vi "OP5_PRESSURIZZAZIONE.vi"(0 "Esito 2 in":cluster{"Si":bool, "No":bool}, 1 "Esito 3 in":cluster{"Si":bool, "No":bool}, 2 "Esito 4 in":cluster{"Si":bool, "No":bool}, 3 "Esito 5 in":cluster{"Si":bool, "No":bool}, 4 "Esito 6 in":cluster{"Si":bool, "No":bool}, 5 "Esito 7 in":cluster{"Si":bool, "No":bool}, 6 "Esito 8 in":cluster{"Si":bool, "No":bool}, 7 "Esito 9 in":cluster{"Si":bool, "No":bool}, 8 "Esito 1 in":cluster{"Si":bool, "No":bool}, 9 "Tasto premuto":T1(array[ring]), 10 "Tipo specifica":string, 12 "Stato in":u16, 14 "Stato out":u16) -> (16 "Dato":string[](array[string]), 17 "ANNULLA PROVA":bool, 18 "Esito 1 out":T2, 19 "i out":i32=1, 20 "Esito 2 out":T2, 21 "Esito 3 out":T2, 22 "Esito 4 out":T2, 23 "Esito 5 out":T2, 24 "Esito 6 out":T2, 25 "Esito 7 out":T2, 26 "Esito 8 out":T2, 27 "Esito 9 out":T2)   [LabVIEW 2022 SP3]
uses:
  Labview/Globali.vi
panel:
  in  "i max":i32
  in  "i":i32=1
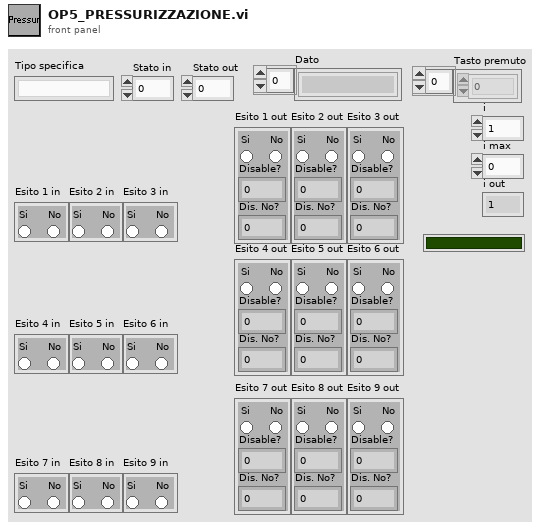
[diagram p1: front panel]
types:
  T1 = enum16{"0", "1", "2", "3", "4", "5", "6", "7", "8", "9", "A", "B", "C", "D", "E", "F", "G", "H", "I", "J", "K", "L", "M", "N", "O", "P", "Q", "R", "S", "T", "U", "V", "W", "X", "Y", "Z", "F1", "F2", "F3", "F4", "F5", "F6", "F7", "F8", "F9", "F10", "F11", "F12", "F13", "F14", "F15", "ADD", "BACK", "BACKSLASH", "CAPITAL", "COMMA", "DECIMAL", "DELETE", "DIVIDE", "DOWN", "END", "EQUALS", "ESCAPE", "GRAVE (`)", "HOME", "INSERT", "LBRACKET", "LCONTROL", "LEFT", "L ALT", "LSHIFT", "LWIN", "MINUS", "MULTIPLY", "NEXT", "NUMLOCK", "NUMPAD_0", "NUMPAD_1", "NUMPAD_2", "NUMPAD_3", "NUMPAD_4", "NUMPAD_5", "NUMPAD_6", "NUMPAD_7", "NUMPAD_8", "NUMPAD_9", "PAUSE", "PERIOD", "PRIOR (PG UP)", "RBRACKET", "RCONTROL", "RETURN", "RIGHT", "R ALT", "RSHIFT", "RWIN", "SCROLL", "SEMICOLON", "SLASH", "SPACE", "SUBTRACT", "TAB", "UP", "ENTER (num pad)", "' (quote)"}[]
  T2 = cluster{"Disable?":i16, "Si":bool, "No":bool, "Dis. No?":i16}
  T3 = cluster{"Esito 1 out":cluster{"Disable?":i16, "Si":bool, "No":bool, "Dis. No?":i16}, "Esito 2 out":cluster{"Disable?":i16, "Si":bool, "No":bool, "Dis. No?":i16}, "Esito 3 out":cluster{"Disable?":i16, "Si":bool, "No":bool, "Dis. No?":i16}, "Esito 4 out":cluster{"Disable?":i16, "Si":bool, "No":bool, "Dis. No?":i16}, "Esito 5 out":cluster{"Disable?":i16, "Si":bool, "No":bool, "Dis. No?":i16}, "Esito 6 out":cluster{"Disable?":i16, "Si":bool, "No":bool, "Dis. No?":i16}, "Esito 7 out":cluster{"Disable?":i16, "Si":bool, "No":bool, "Dis. No?":i16}, "Esito 8 out":cluster{"Disable?":i16, "Si":bool, "No":bool, "Dis. No?":i16}, "Esito 9 out":cluster{"Disable?":i16, "Si":bool, "No":bool, "Dis. No?":i16}}
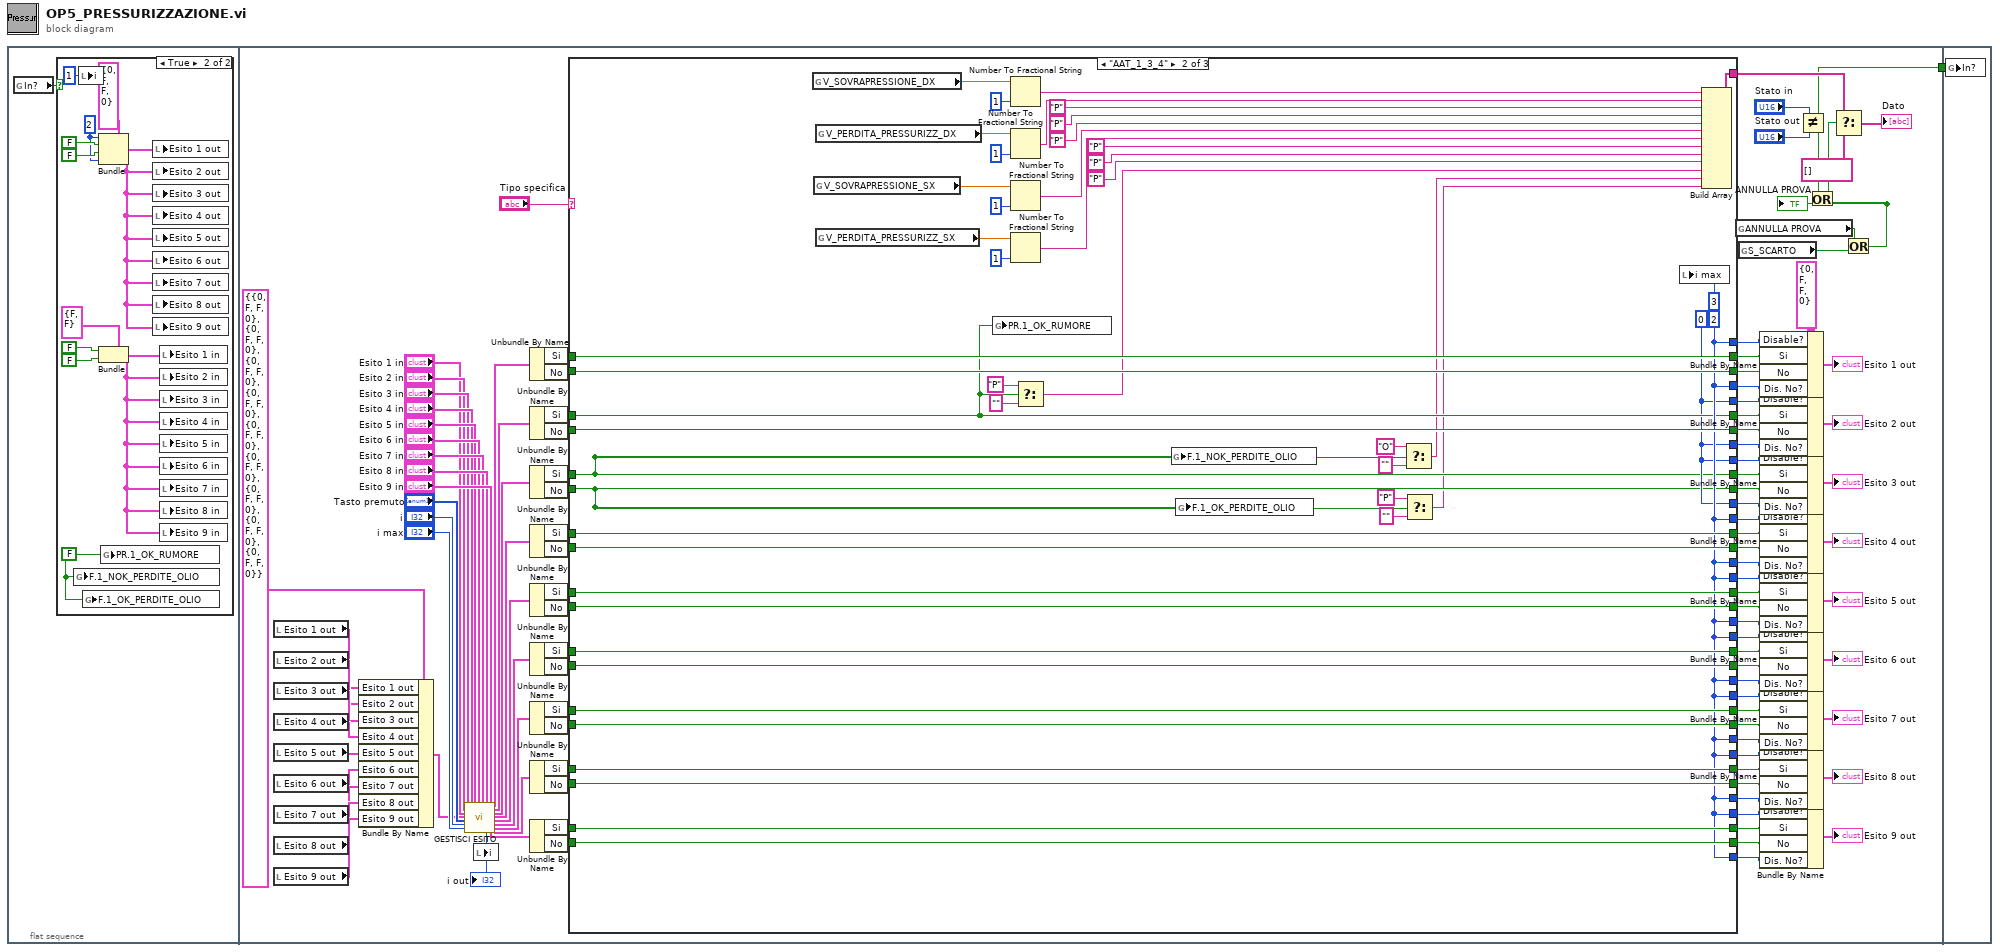
[diagram p0: block diagram]
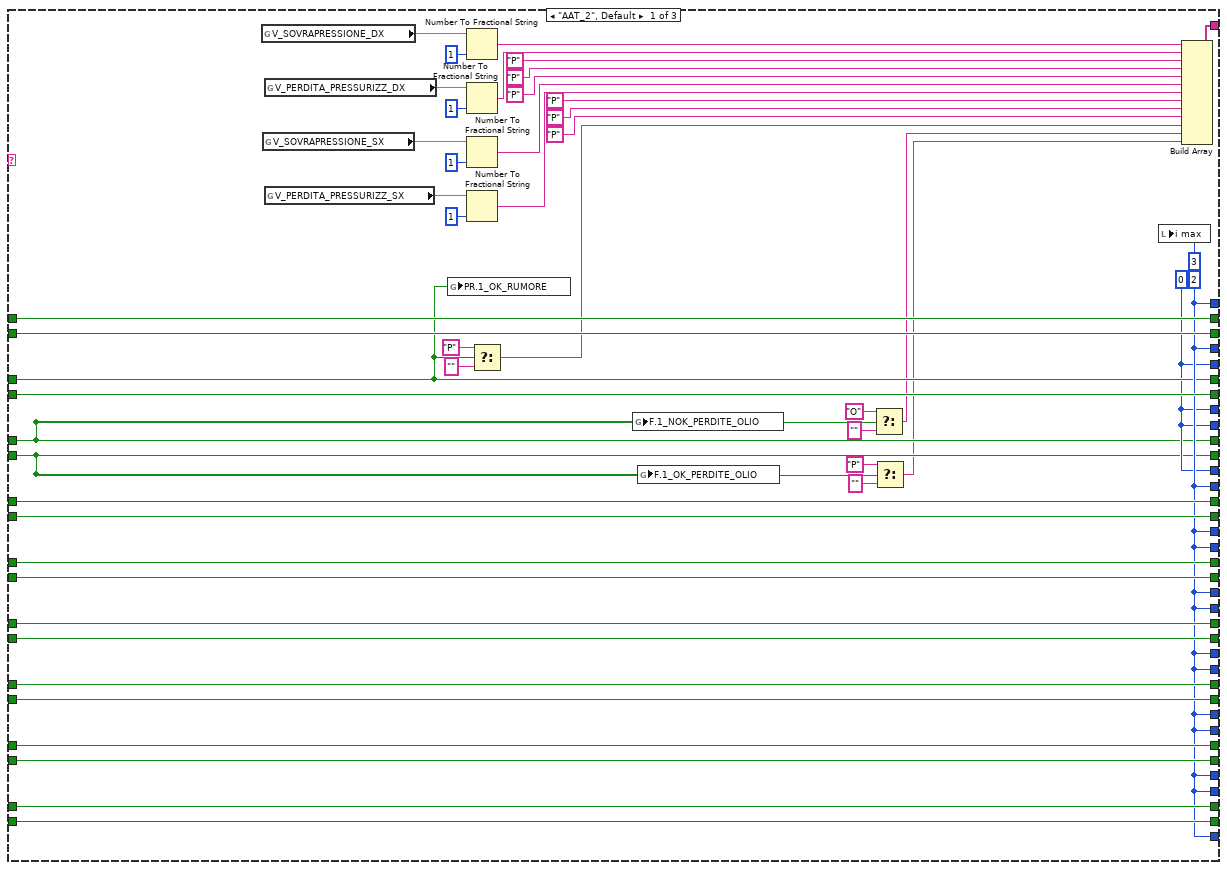
[diagram p3: hidden frame]
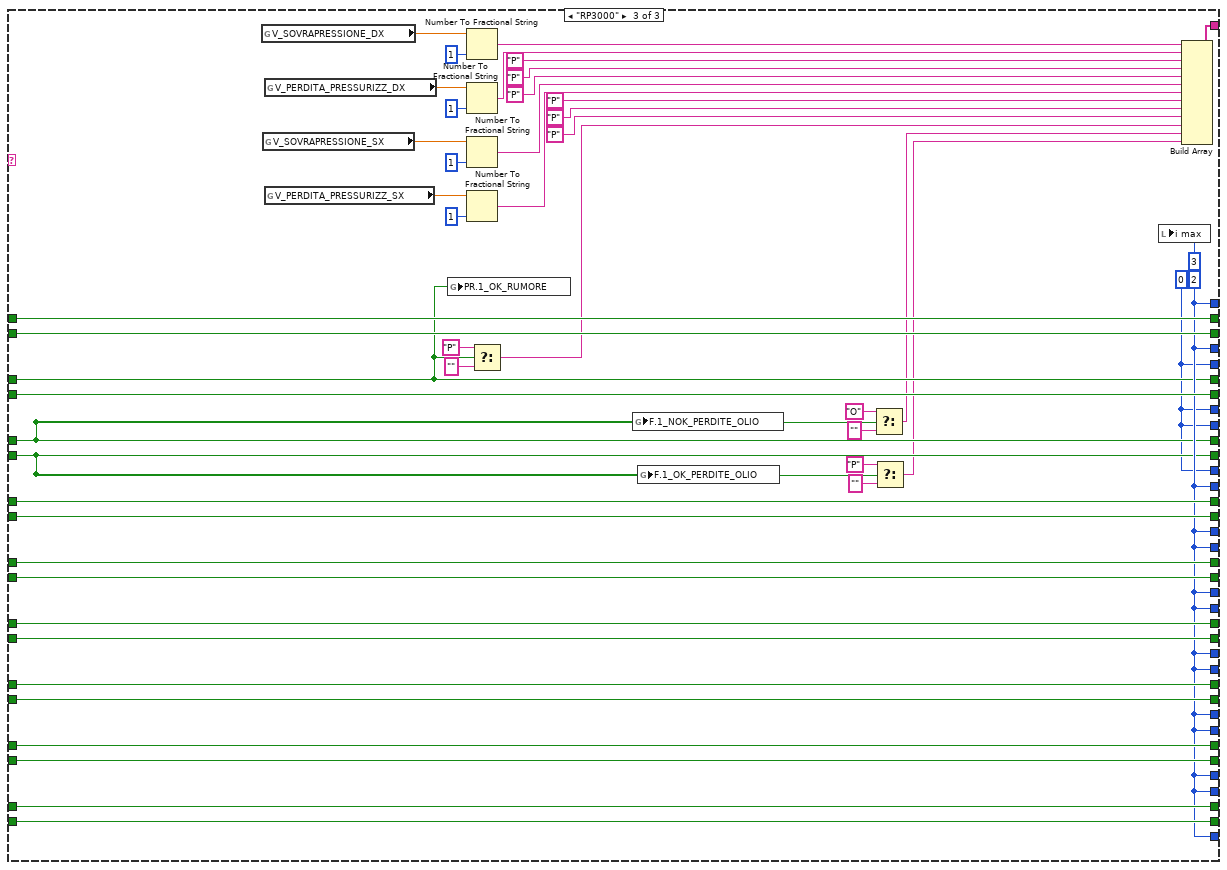
[diagram p4: hidden frame]
diagram:
  n1 = flat-sequence {
    tunnel: [w18] -> w1
    tunnel: w1 -> [w269]
    frame #0 {
      n2 = global read "Globali.vi" "In?"() -> (w2:bool)
      n3 = case shown="True" w2 {
        frame False {
        }
        frame True {
          w3 = FALSE ("No")
          w10 = i16 2 ("Disable?")
          n4 = global write "Globali.vi" "F.1_NOK_PERDITE_OLIO"(w3) -> ()
          n5 = local write "i"(1 ("i")) -> ()
          n6 = global write "Globali.vi" "F.1_OK_PERDITE_OLIO"(w3) -> ()
          n7 = Bundle(cluster=T2 {"Disable?"=0, "Si"=FALSE, "No"=FALSE, "Dis. No?"=0} ("Esito 1 out"), "Disable?"=w10, "Si"=FALSE, "No"=FALSE, "Dis. No?"=w10) -> (w9:T2)
          n8 = Bundle(cluster=cluster{"Si":bool, "No":bool} {"Si"=FALSE, "No"=FALSE} ("Esito 1 in"), "Si"=FALSE, "No"=FALSE) -> (w7:cluster{"Si":bool, "No":bool})
          n9 = global write "Globali.vi" "PR.1_OK_RUMORE"(w3) -> ()
          n10 = local write "Esito 1 out"(w9) -> ()
          n11 = local write "Esito 2 out"(w9) -> ()
          n12 = local write "Esito 3 out"(w9) -> ()
          n13 = local write "Esito 4 out"(w9) -> ()
          n14 = local write "Esito 5 out"(w9) -> ()
          n15 = local write "Esito 6 out"(w9) -> ()
          n16 = local write "Esito 7 out"(w9) -> ()
          n17 = local write "Esito 8 out"(w9) -> ()
          n18 = local write "Esito 9 out"(w9) -> ()
          n19 = local write "Esito 1 in"(w7) -> ()
          n20 = local write "Esito 2 in"(w7) -> ()
          n21 = local write "Esito 3 in"(w7) -> ()
          n22 = local write "Esito 4 in"(w7) -> ()
          n23 = local write "Esito 5 in"(w7) -> ()
          n24 = local write "Esito 6 in"(w7) -> ()
          n25 = local write "Esito 7 in"(w7) -> ()
          n26 = local write "Esito 8 in"(w7) -> ()
          n27 = local write "Esito 9 in"(w7) -> ()
        }
      }
    }
    frame #1 {
      w61 = T2 {"Disable?"=0, "Si"=FALSE, "No"=FALSE, "Dis. No?"=0} ("Esito 1 out")
      n28 = local read "Esito 1 out"() -> (w39:T2)
      n29 = local read "Esito 2 out"() -> (w40:T2)
      n30 = local read "Esito 3 out"() -> (w41:T2)
      n31 = local read "Esito 4 out"() -> (w42:T2)
      n32 = local read "Esito 5 out"() -> (w43:T2)
      n33 = local read "Esito 6 out"() -> (w44:T2)
      n34 = local read "Esito 7 out"() -> (w45:T2)
      n35 = local read "Esito 8 out"() -> (w46:T2)
      n36 = local read "Esito 9 out"() -> (w47:T2)
      n37 = Bundle By Name(cluster=T3 {"Esito 1 out"={"Disable?"=0, "Si"=FALSE, "No"=FALSE, "Dis. No?"=0}, "Esito 2 out"={"Disable?"=0, "Si"=FALSE, "No"=FALSE, "Dis. No?"=0}, "Esito 3 out"={"Disable?"=0, "Si"=FALSE, "No"=FALSE, "Dis. No?"=0}, "Esito 4 out"={"Disable?"=0, "Si"=FALSE, "No"=FALSE, "Dis. No?"=0}, "Esito 5 out"={"Disable?"=0, "Si"=FALSE, "No"=FALSE, "Dis. No?"=0}, "Esito 6 out"={"Disable?"=0, "Si"=FALSE, "No"=FALSE, "Dis. No?"=0}, "Esito 7 out"={"Disable?"=0, "Si"=FALSE, "No"=FALSE, "Dis. No?"=0}, "Esito 8 out"={"Disable?"=0, "Si"=FALSE, "No"=FALSE, "Dis. No?"=0}, "Esito 9 out"={"Disable?"=0, "Si"=FALSE, "No"=FALSE, "Dis. No?"=0}} ("Cluster"), "Esito 1 out"=w39, "Esito 2 out"=w40, "Esito 3 out"=w41, "Esito 4 out"=w42, "Esito 5 out"=w43, "Esito 6 out"=w44, "Esito 7 out"=w45, "Esito 8 out"=w46, "Esito 9 out"=w47) -> (w48:T3)
      n38 = call "GESTISCI ESITO.vi"("Esito 3 in"="Esito 3 in", "Esito 2 in"="Esito 2 in", "Esito 1 in"="Esito 1 in", "Cluster"=w48, "Tasto premuto"="Tasto premuto", "i in"="i", "i max"="i max", "Esito 4 in"="Esito 4 in", "Esito 5 in"="Esito 5 in", "Esito 6 in"="Esito 6 in", "Esito 7 in"="Esito 7 in", "Esito 8 in"="Esito 8 in", "Esito 9 in"="Esito 9 in") -> ("i out"=w19:i32, "Esito 9 in 2"=w37:cluster{"Si":bool, "No":bool}, "Esito 1 in 2"=w29:cluster{"Si":bool, "No":bool}, "Esito 2 in 2"=w30:cluster{"Si":bool, "No":bool}, "Esito 3 in 2"=w31:cluster{"Si":bool, "No":bool}, "Esito 4 in 2"=w32:cluster{"Si":bool, "No":bool}, "Esito 5 in 2"=w33:cluster{"Si":bool, "No":bool}, "Esito 6 in 2"=w34:cluster{"Si":bool, "No":bool}, "Esito 7 in 2"=w36:cluster{"Si":bool, "No":bool}, "Esito 8 in 2"=w35:cluster{"Si":bool, "No":bool})  [unwired: 5 in]
      "i out" <- w19
      n39 = local write "i"(w19) -> ()
      n40 = Unbundle By Name(w29) -> ("Si"=w85:bool, "No"=w84:bool)
      n41 = Unbundle By Name(w30) -> ("Si"=w68:bool, "No"=w69:bool)
      n42 = Unbundle By Name(w31) -> ("Si"=w70:bool, "No"=w71:bool)
      n43 = Unbundle By Name(w32) -> ("Si"=w72:bool, "No"=w73:bool)
      n44 = Unbundle By Name(w33) -> ("Si"=w74:bool, "No"=w75:bool)
      n45 = Unbundle By Name(w34) -> ("Si"=w76:bool, "No"=w77:bool)
      n46 = Unbundle By Name(w36) -> ("Si"=w78:bool, "No"=w79:bool)
      n47 = Unbundle By Name(w35) -> ("Si"=w80:bool, "No"=w81:bool)
      n48 = Unbundle By Name(w37) -> ("Si"=w82:bool, "No"=w83:bool)
      n49 = case shown="\"AAT_1_3_4\"" "Tipo specifica" {
        tunnel: [w148 w193 w246] -> w65
        tunnel: [w155 w204 w253] -> w112
        tunnel: [w130 w179 w224] -> w111
        tunnel: [w130 w179 w224] -> w110
        tunnel: [w155 w204 w253] -> w109
        tunnel: [w155 w204 w253] -> w108
        tunnel: [w155 w204 w253] -> w107
        tunnel: [w155 w204 w253] -> w106
        tunnel: [w155 w204 w253] -> w105
        tunnel: [w155 w204 w253] -> w104
        tunnel: [w156 w205 w254] -> w103
        tunnel: [w161 w210 w259] -> w102
        tunnel: [w131 w180 w233] -> w101
        tunnel: [w162 w211 w260] -> w100
        tunnel: [w125 w174 w228] -> w99
        tunnel: [w124 w173 w227] -> w98
        tunnel: [w157 w206 w255] -> w97
        tunnel: [w170 w219 w268] -> w96
        tunnel: [w160 w209 w258] -> w95
        tunnel: [w169 w218 w267] -> w94
        tunnel: [w159 w208 w257] -> w93
        tunnel: [w168 w217 w266] -> w92
        tunnel: [w158 w207 w256] -> w91
        tunnel: [w167 w216 w265] -> w90
        tunnel: [w166 w215 w264] -> w89
        tunnel: [w165 w214 w263] -> w88
        tunnel: [w164 w213 w262] -> w87
        tunnel: [w163 w212 w261] -> w86
        tunnel: w85 -> [w156 w205 w254]
        tunnel: w84 -> [w161 w210 w259]
        tunnel: w83 -> [w163 w212 w261]
        tunnel: w82 -> [w164 w213 w262]
        tunnel: w81 -> [w165 w214 w263]
        tunnel: w80 -> [w166 w215 w264]
        tunnel: w79 -> [w167 w216 w265]
        tunnel: w78 -> [w158 w207 w256]
        tunnel: w77 -> [w168 w217 w266]
        tunnel: w76 -> [w159 w208 w257]
        tunnel: w75 -> [w169 w218 w267]
        tunnel: w74 -> [w160 w209 w258]
        tunnel: w73 -> [w170 w219 w268]
        tunnel: w72 -> [w157 w206 w255]
        tunnel: w71 -> [w124 w173 w227]
        tunnel: w70 -> [w125 w174 w228]
        tunnel: w69 -> [w162 w211 w260]
        tunnel: w68 -> [w131 w180 w233]
        tunnel: [w155 w204 w253] -> w60
        tunnel: [w130 w179 w224] -> w59
        tunnel: [w130 w179 w224] -> w58
        tunnel: [w155 w204 w253] -> w57
        tunnel: [w155 w204 w253] -> w56
        tunnel: [w155 w204 w253] -> w55
        tunnel: [w155 w204 w253] -> w54
        tunnel: [w155 w204 w253] -> w53
        tunnel: [w155 w204 w253] -> w52
        frame "AAT_2", Default {
          w155 = 2
          w130 = 0
          n50 = global read "Globali.vi" "V_SOVRAPRESSIONE_DX"() -> (w135:sgl)
          n51 = global read "Globali.vi" "V_SOVRAPRESSIONE_SX"() -> (w133:sgl)
          n52 = global read "Globali.vi" "V_PERDITA_PRESSURIZZ_DX"() -> (w134:sgl)
          n53 = global read "Globali.vi" "V_PERDITA_PRESSURIZZ_SX"() -> (w132:sgl)
          n54 = global write "Globali.vi" "PR.1_OK_RUMORE"(w131) -> ()
          n55 = Number To Fractional String(number=w135, precision (6)=i16 1) -> (F-format string=w147:string)  [unwired: 2 in]
          n56 = Number To Fractional String(number=w134, precision (6)=i16 1) -> (F-format string=w146:string)  [unwired: 2 in]
          n57 = Number To Fractional String(number=w133, precision (6)=i16 1) -> (F-format string=w142:string)  [unwired: 2 in]
          n58 = Number To Fractional String(number=w132, precision (6)=i16 1) -> (F-format string=w141:string)  [unwired: 2 in]
          n59 = Select(t="P", s=w131, f="") -> (s? t:f=w137:string)
          n60 = global write "Globali.vi" "F.1_NOK_PERDITE_OLIO"(w125) -> ()
          n61 = global write "Globali.vi" "F.1_OK_PERDITE_OLIO"(w124) -> ()
          n62 = Select(t="O", s=w125, f="") -> (s? t:f=w123:string)
          n63 = Select(t="P", s=w124, f="") -> (s? t:f=w122:string)
          n64 = local write "i max"(3) -> ()
          n65 = Build Array(w147, w146, "P", "P", "P", w142, w141, "P", "P", "P", w137, w123, w122) -> (w148:string[])
        }
        frame "AAT_1_3_4" {
          w204 = 2
          w179 = 0
          n66 = global read "Globali.vi" "V_SOVRAPRESSIONE_DX"() -> (w199:sgl)
          n67 = global read "Globali.vi" "V_SOVRAPRESSIONE_SX"() -> (w196:sgl)
          n68 = global read "Globali.vi" "V_PERDITA_PRESSURIZZ_DX"() -> (w198:sgl)
          n69 = global read "Globali.vi" "V_PERDITA_PRESSURIZZ_SX"() -> (w197:sgl)
          n70 = global write "Globali.vi" "PR.1_OK_RUMORE"(w180) -> ()
          n71 = Number To Fractional String(number=w199, precision (6)=i16 1) -> (F-format string=w192:string)  [unwired: 2 in]
          n72 = Number To Fractional String(number=w198, precision (6)=i16 1) -> (F-format string=w191:string)  [unwired: 2 in]
          n73 = Number To Fractional String(number=w196, precision (6)=i16 1) -> (F-format string=w187:string)  [unwired: 2 in]
          n74 = Number To Fractional String(number=w197, precision (6)=i16 1) -> (F-format string=w186:string)  [unwired: 2 in]
          n75 = Select(t="P", s=w180, f="") -> (s? t:f=w182:string)
          n76 = global write "Globali.vi" "F.1_NOK_PERDITE_OLIO"(w174) -> ()
          n77 = global write "Globali.vi" "F.1_OK_PERDITE_OLIO"(w173) -> ()
          n78 = Select(t="O", s=w174, f="") -> (s? t:f=w172:string)
          n79 = Select(t="P", s=w173, f="") -> (s? t:f=w171:string)
          n80 = local write "i max"(3) -> ()
          n81 = Build Array(w192, w191, "P", "P", "P", w187, w186, "P", "P", "P", w182, w172, w171) -> (w193:string[])
        }
        frame "RP3000" {
          w253 = 2
          w224 = 0
          n82 = global read "Globali.vi" "V_SOVRAPRESSIONE_DX"() -> (w221:sgl)
          n83 = global read "Globali.vi" "V_SOVRAPRESSIONE_SX"() -> (w220:sgl)
          n84 = global read "Globali.vi" "V_PERDITA_PRESSURIZZ_DX"() -> (w222:sgl)
          n85 = global read "Globali.vi" "V_PERDITA_PRESSURIZZ_SX"() -> (w223:sgl)
          n86 = global write "Globali.vi" "PR.1_OK_RUMORE"(w233) -> ()
          n87 = Number To Fractional String(number=w221, precision (6)=i16 1) -> (F-format string=w245:string)  [unwired: 2 in]
          n88 = Number To Fractional String(number=w222, precision (6)=i16 1) -> (F-format string=w244:string)  [unwired: 2 in]
          n89 = Number To Fractional String(number=w220, precision (6)=i16 1) -> (F-format string=w240:string)  [unwired: 2 in]
          n90 = Number To Fractional String(number=w223, precision (6)=i16 1) -> (F-format string=w239:string)  [unwired: 2 in]
          n91 = Select(t="P", s=w233, f="") -> (s? t:f=w235:string)
          n92 = global write "Globali.vi" "F.1_NOK_PERDITE_OLIO"(w228) -> ()
          n93 = global write "Globali.vi" "F.1_OK_PERDITE_OLIO"(w227) -> ()
          n94 = Select(t="O", s=w228, f="") -> (s? t:f=w226:string)
          n95 = Select(t="P", s=w227, f="") -> (s? t:f=w225:string)
          n96 = local write "i max"(3) -> ()
          n97 = Build Array(w245, w244, "P", "P", "P", w240, w239, "P", "P", "P", w235, w226, w225) -> (w246:string[])
        }
      }
      n98 = global read "Globali.vi" "ANNULLA PROVA"() -> (w16:bool)
      n99 = global read "Globali.vi" "S_SCARTO"() -> (w15:bool)
      n100 = Bundle By Name(cluster=w61, "Disable?"=w112, "Si"=w103, "No"=w102, "Dis. No?"=w60) -> (→"Esito 1 out":T2)
      n101 = Bundle By Name(cluster=w61, "Disable?"=w111, "Si"=w101, "No"=w100, "Dis. No?"=w59) -> (→"Esito 2 out":T2)
      n102 = Bundle By Name(cluster=w61, "Disable?"=w110, "Si"=w99, "No"=w98, "Dis. No?"=w58) -> (→"Esito 3 out":T2)
      n103 = Bundle By Name(cluster=w61, "Disable?"=w109, "Si"=w97, "No"=w96, "Dis. No?"=w57) -> (→"Esito 4 out":T2)
      n104 = Bundle By Name(cluster=w61, "Disable?"=w108, "Si"=w95, "No"=w94, "Dis. No?"=w56) -> (→"Esito 5 out":T2)
      n105 = Bundle By Name(cluster=w61, "Disable?"=w107, "Si"=w93, "No"=w92, "Dis. No?"=w55) -> (→"Esito 6 out":T2)
      n106 = Bundle By Name(cluster=w61, "Disable?"=w106, "Si"=w91, "No"=w90, "Dis. No?"=w54) -> (→"Esito 7 out":T2)
      n107 = Bundle By Name(cluster=w61, "Disable?"=w105, "Si"=w89, "No"=w88, "Dis. No?"=w53) -> (→"Esito 8 out":T2)
      n108 = Bundle By Name(cluster=w61, "Disable?"=w104, "Si"=w87, "No"=w86, "Dis. No?"=w52) -> (→"Esito 9 out":T2)
      n109 = Not Equal?(x="Stato in", y="Stato out") -> (x != y?=w18:bool)
      n110 = Or(x=w16, y=w15) -> (x .or. y?=w14:bool)
      "ANNULLA PROVA" <- w14
      n111 = Or(x=w18, y=w14) -> (x .or. y?=w17:bool)
      n112 = Select(t=w65, s=w17, f=string[] [] ("Dato")) -> (s? t:f=→"Dato":string[])
    }
    frame #2 {
      n113 = global write "Globali.vi" "In?"(w269) -> ()
    }
  }
